vi "MainGui-StatusMsgUpdate2.vi"(6 "Blink":bool, 7 "Arguments":variant[](array[variant]), 8 "error in (no error)":errorcluster, 9 "TxtColor":u32(colorbox), 10 "BgColor":u32(colorbox)=13816530, 11 "Msg":T1) -> (0 "error out":errorcluster)   [LabVIEW 2016]
uses:
  Tools/Translator/Translator.Message.ctl
  MainGui.UserMsg.ctl
  MainGui.Action.ctl
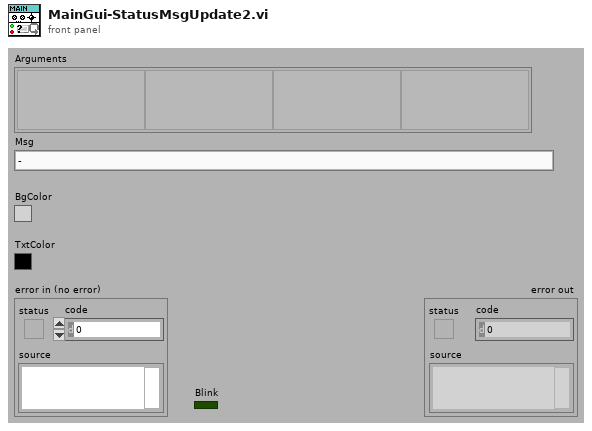
[diagram p1: front panel]
types:
  T1 = typedef "Translator.Message.ctl" = enum16{"-", "Event confirmed", "Log out", "Log in", "Shutdown", "Cancel", "Start", "Continue", "Stop", "On", "Off", "OK", "NOK", "NOK %s", "Home", "Work", "In progress...", "Missing", "Empty", "Hardware failure", "Initial", "Error %d >> %s", "Error %d >> %s >> %s", "Starting %s", "Quitting %s", "Configured", "Initializing", "Quitting", "Loading", "Running %s", "Stopped", "Summary", "Do you want to continue?", "Do you want to exit?", "Log out?", "System", "All", "IDLE", "Translating...%s", "Not found", "Alarm %s", "Run", "Skip", "Abort", "Repeat", "Please wait...", "Database disconnected", "Database disconnected - changeover disabled!", "Login to database successful", "Login to database failed: %d; %s", "Read steps (%s)", "Result A", "Result B", "Unkown reference", "Msg %d >> %s", "PLC LifeBit Failure", "Reconnecting database"}
  T2 = typedef "MainGui.UserMsg.ctl" = cluster{"Msg":T1, "Arguments":variant[], "BgColor":u32, "TxtColor":u32, "Blink":bool}
  T3 = typedef "MainGui.Action.ctl" = enum32{"idle", "constructor", "destructor", "--- MainGui ---", "Error.Update", "Error.Confirm", "TopBar.Update", "Buttons.Update", "StatusMsg.Update", "StatusTable.Update"}
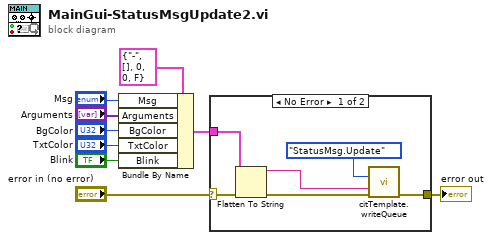
[diagram p0: block diagram]
diagram:
  n1 = Bundle By Name(cluster=T2 {"Msg"=enum."-", "Arguments"=[], "BgColor"=0, "TxtColor"=0, "Blink"=FALSE} ("UsrMsg"), "Msg"="Msg", "Arguments"="Arguments", "BgColor"="BgColor", "TxtColor"="TxtColor", "Blink"="Blink") -> (w3:T2)
  n2 = case shown="No Error" "error in (no error)" {
    selector: "error in (no error)" -> [w13 w16]
    tunnel: [w15 w16] -> w8
    tunnel: w3 -> [w11 _]
    frame No Error {
      n3 = Flatten To String(anything=w11, error in (no error)=w13) -> (data string=w10:string, error out=w12:errorcluster)  [unwired: 2 in, 1 out]
      n4 = call "citTemplate.writeQueue.vi"("event in (if not connected:all statemachine with data event)"=MainGui.Action."StatusMsg.Update" ("Action"), "data in"=w10, "error in (no error)"=w12) -> ("error out"=w15:errorcluster)  [unwired: 12 in]
    }
    frame Error {
    }
  }
  "error out" <- w8
